vi "DRAFT5.vi"() -> ()   [LabVIEW 2021]
uses:
  e66af977-9b25-48cf-95ca-2a006889b648.vi
  <vilib>/Analysis/3filter.llb/Butterworth Filter (DBL).vi
  <vilib>/Analysis/NI_AALBase.lvlib
  <vilib>/ptbypt/NI_PtbyPt.lvlib
panel:
  in  "Boolean 2":bool
  out "Waveform Graph 7":dynamicdata(graph)
  out "Array Size 2":u32
  out "Array Size":u32
  out "Elapsed time in ms":u32
  in  "stop":bool
  in  "error in (no error)":errorcluster
  out "error out":errorcluster
  in  "loop 1":i32
  out "Waveform Graph 6":dynamicdata(graph)
  out "Waveform Graph 5":dynamicdata(graph)
  out "Waveform Graph 4":dynamicdata(graph)
  out "Waveform Graph 3":dbl[](graph)
  out "Waveform Graph 2":dynamicdata(graph)
  in  "Boolean":bool
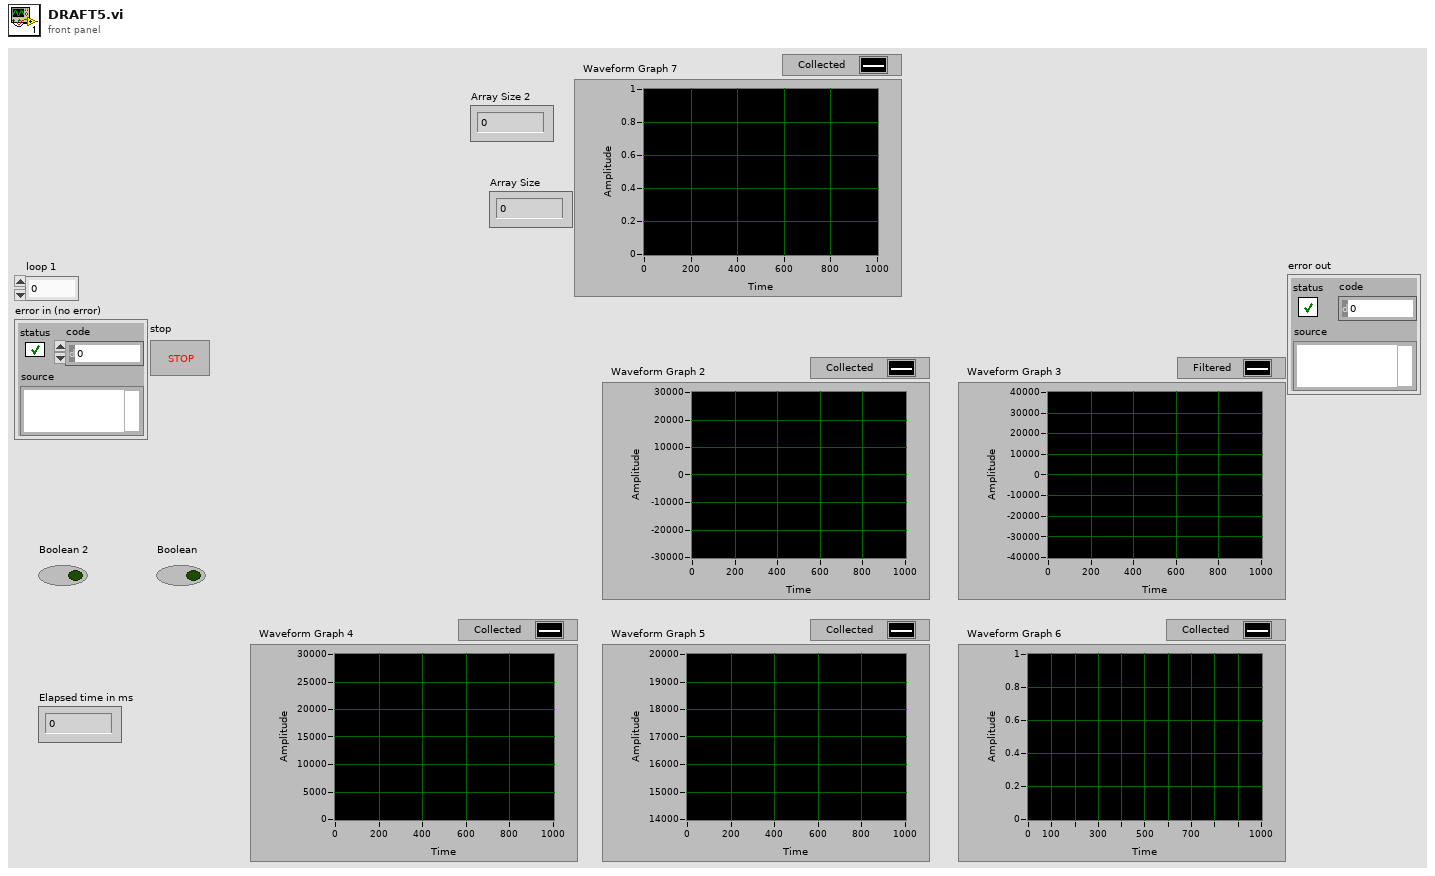
[diagram p1: front panel]
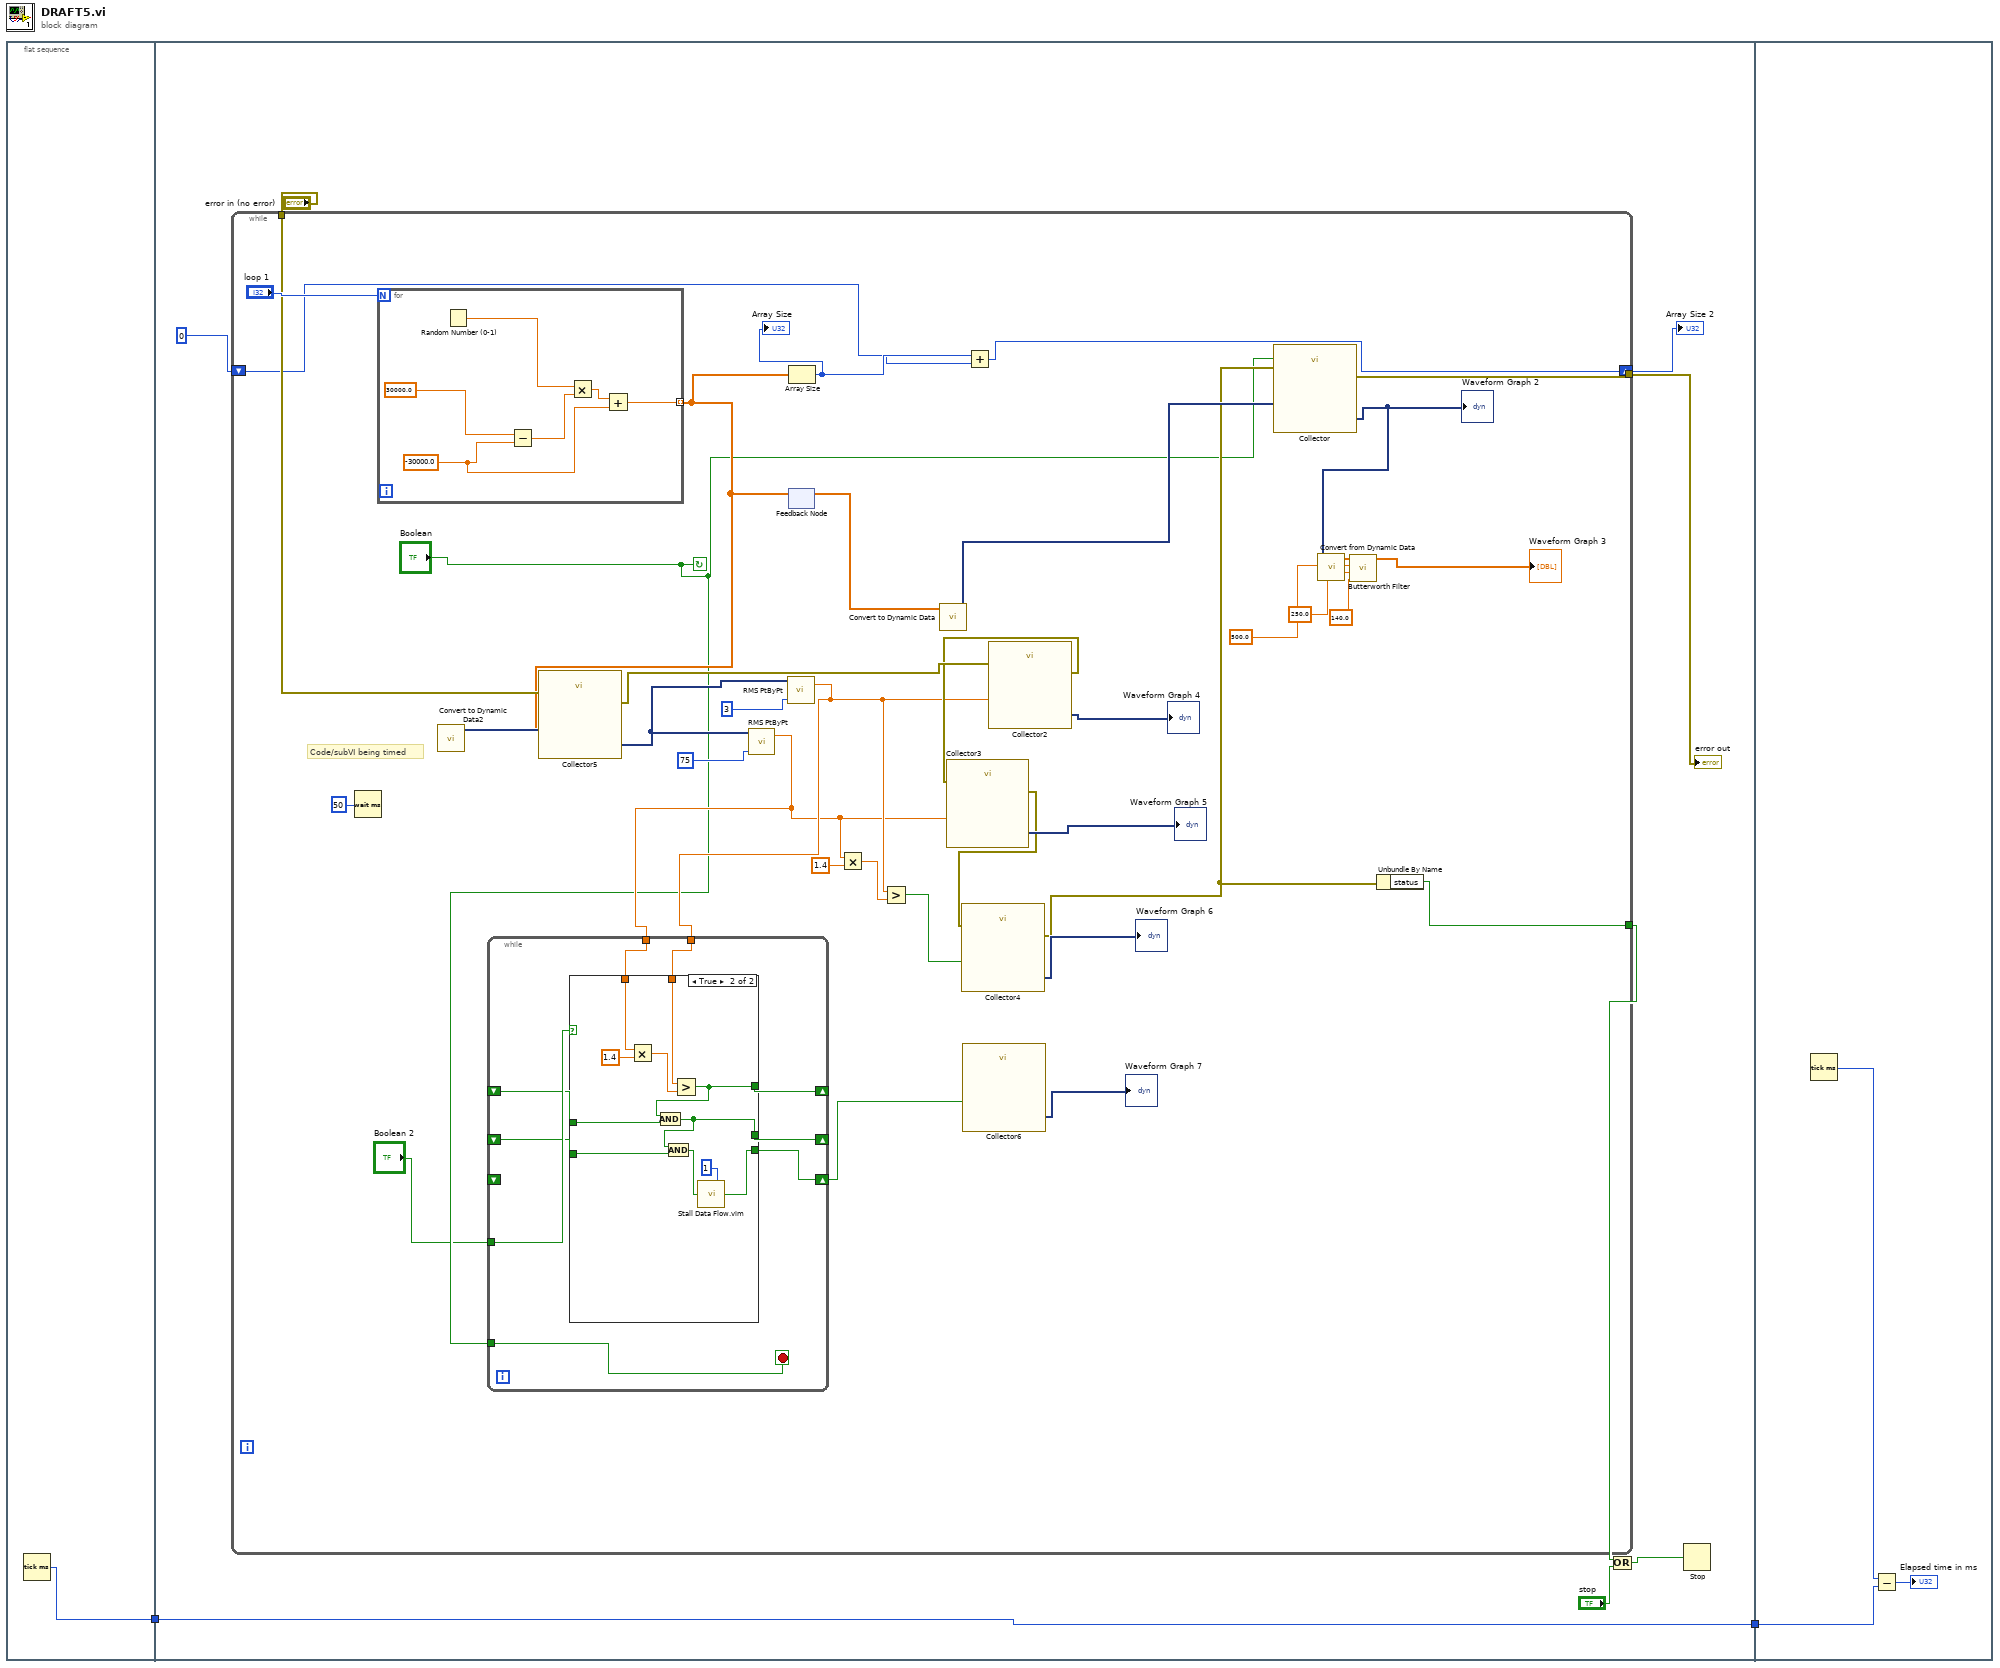
[diagram p0: block diagram]
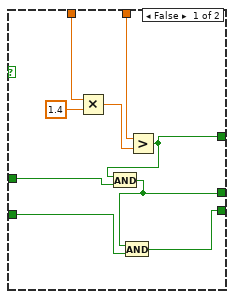
[diagram p2: hidden frame]
diagram:
  n1 = flat-sequence {
    tunnel: [w3] -> w2
    tunnel: [w12] -> w1
    tunnel: w2 -> [w12]
    tunnel: w1 -> [w84]
    frame #0 {
      n2 = Tick Count (ms)() -> (millisecond timer value=w3:u32)
    }
    frame #1 {
      # "Code/subVI being timed"
      n3 = while {
        tunnel: "error in (no error)" -> [w30]
        tunnel: [w26] -> w9
        tunnel: [w24] -> w8
        shift-right: [w19] -> w4
        shift-left: 0 -> [w20]
        stop <- "Boolean" continue-if-true
        n4 = for {
          N: "loop 1" -> [_]
          tunnel: [w78] -> w22 mode=indexing
          w80 = -30000.0 ("y")
          n5 = Random Number (0-1)() -> (number: 0 to 1=w79:dbl)
          n6 = Subtract(x=30000.0, y=w80) -> (x-y=w83:dbl)
          n7 = Multiply(x=w79, y=w83) -> (x*y=w82:dbl)
          n8 = Add(x=w82, y=w80) -> (x+y=w78:dbl)
        }
        n9 = call "Convert to Dynamic Data2"("Array"=w22) -> ("Dynamic Data Type"=w32:dynamicdata)  [unwired: 3 in]
        n10 = call "Collector5"("error in (no error)"=w30, "Signals"=w32) -> ("error out"=w29:errorcluster, "Collected Signals"=w31:dynamicdata)  [unwired: 8 in]
        n11 = call <vilib>:"RMS PtByPt.vi"("sample length"=75, "x"=w31) -> ("rms value"=w16:dbl)  [unwired: 2 in, 1 out]
        n12 = call <vilib>:"RMS PtByPt.vi"("sample length"=3, "x"=w31) -> ("rms value"=w17:dbl)  [unwired: 2 in, 1 out]
        n13 = while {
          tunnel: w17 -> [w53]
          tunnel: w16 -> [w54]
          shift-right: [w49] -> _
          shift-left: _ -> [w56]
          shift-right: [w52] -> _
          shift-left: _ -> [w55]
          tunnel: "Boolean" -> [w51]
          shift-right: [w50] -> w14
          shift-left: _ -> [_]
          tunnel: "Boolean 2" -> [w57]
          stop <- w51 stop-if-true
          n14 = case shown="True" w57 {
            tunnel: w56 -> [w63 w76]
            tunnel: w55 -> [w64 w75]
            tunnel: w54 -> [w62 w73]
            tunnel: w53 -> [w61 w72]
            tunnel: [w59 w71] -> w49
            tunnel: [w58 w70] -> w52
            tunnel: [w60 w68] -> w50
            frame False {
              n15 = Multiply(x=w62, y=1.4) -> (x*y=w66:dbl)
              n16 = Greater?(x=w61, y=w66) -> (0:w58:bool)
              n17 = And(x=w58, y=w64) -> (x .and. y?=w59:bool)
              n18 = And(x=w59, y=w63) -> (x .and. y?=w60:bool)
            }
            frame True {
              n19 = Multiply(x=w73, y=1.4) -> (x*y=w77:dbl)
              n20 = Greater?(x=w72, y=w77) -> (0:w70:bool)
              n21 = And(x=w70, y=w75) -> (x .and. y?=w71:bool)
              n22 = And(x=w71, y=w76) -> (x .and. y?=w69:bool)
              n23 = call "Stall Data Flow.vim"("value in"=w69, "milliseconds to wait"=u32 1) -> ("value out"=w68:bool)  [unwired: 1 out]
            }
          }
        }
        n24 = feedback-in #1(w22) -> ()
        n25 = feedback #1() -> (w23:dbl[])  [unwired: 1 in]
        n26 = Array Size(array=w22) -> (size(s)=w21:i32)
        "Array Size" <- w21
        n27 = Multiply(x=w16, y=1.4) -> (x*y=w36:dbl)
        n28 = Greater?(x=w17, y=w36) -> (0:w35:bool)
        n29 = call "Convert to Dynamic Data"("Array"=w23) -> ("Dynamic Data Type"=w40:dynamicdata)  [unwired: 3 in]
        n30 = call "Collector6"("Signals"=w14) -> ("Collected Signals"=→"Waveform Graph 7":dynamicdata)  [unwired: 9 in, 1 out]
        n31 = Add(x=w21, y=w20) -> (x+y=w19:i32)
        n32 = call "Collector2"("error in (no error)"=w29, "Signals"=w17) -> ("error out"=w28:errorcluster, "Collected Signals"=→"Waveform Graph 4":dynamicdata)  [unwired: 8 in]
        n33 = call "Collector3"("error in (no error)"=w28, "Signals"=w16) -> ("error out"=w27:errorcluster, "Collected Signals"=→"Waveform Graph 5":dynamicdata)  [unwired: 8 in]
        n34 = call "Collector4"("error in (no error)"=w27, "Signals"=w35) -> ("error out"=w25:errorcluster, "Collected Signals"=→"Waveform Graph 6":dynamicdata)  [unwired: 8 in]
        n35 = call "Collector"("error in (no error)"=w25, "Enable"="Boolean", "Signals"=w40) -> ("error out"=w26:errorcluster, "Collected Signals"=w43:dynamicdata)  [unwired: 7 in]
        "Waveform Graph 2" <- w43
        n36 = call "Convert from Dynamic Data"("Dynamic Data Type"=w43) -> ("Array"=w45:dbl[])  [unwired: 3 in]
        n37 = call-poly <vilib>:"Butterworth Filter.vi"("low cutoff freq: fl"=140.0, "high cutoff freq: fh"=250.0, "sampling freq: fs"=500.0, "X"=w45) -> ("Filtered X"=→"Waveform Graph 3":dbl[])  [unwired: 4 in, 1 out]
        n38 = Unbundle By Name(w25) -> ("status"=w24:bool)
      }
      "error out" <- w9
      "Array Size 2" <- w4
      n39 = Wait (ms)(milliseconds to wait=u32 50) -> ()  [unwired: 1 out]
      n40 = Or(x=w8, y="stop") -> (x .or. y?=w6:bool)
      n41 = Stop(stop? (T)=w6) -> ()
    }
    frame #2 {
      n42 = Tick Count (ms)() -> (millisecond timer value=w86:u32)
      n43 = Subtract(x=w86, y=w84) -> (x-y=→"Elapsed time in ms":u32)
    }
  }
